vi "Exercise1.8-Dynamic Data.vi"() -> ()   [LabVIEW 2013]
panel:
  out "Waveform Graph":waveform(dbl)(graph)
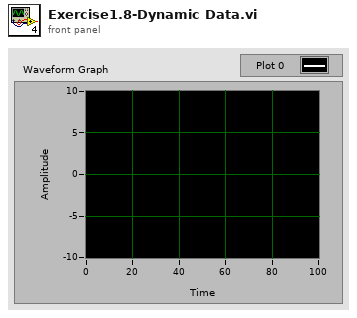
[diagram p1: front panel]
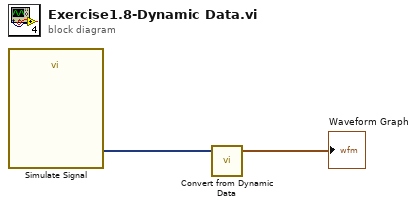
[diagram p0: block diagram]
diagram:
  n1 = call "Simulate Signal"() -> ("Sine"=w2:dynamicdata)  [unwired: 14 in, 1 out]
  n2 = call "Convert from Dynamic Data"("Dynamic Data Type"=w2) -> ("Waveform"=→"Waveform Graph":waveform(dbl))  [unwired: 3 in]
